vi "CreateOrOpenProject.vi"(8 "error in (no error)":errorcluster, 11 "ProjectPath":path) -> (0 "error out":errorcluster)   [LabVIEW 2013, in "ProjectHandler.lvlib"]
uses:
  ProjectHandler.lvlib
  RefNums.vi
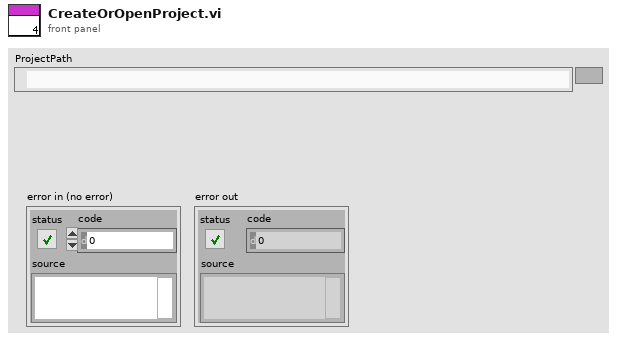
[diagram p1: front panel]
types:
  T1 = cluster{"App":refnum<vi>, "Project":refnum<vi>, "My Computer":refnum<vi>}
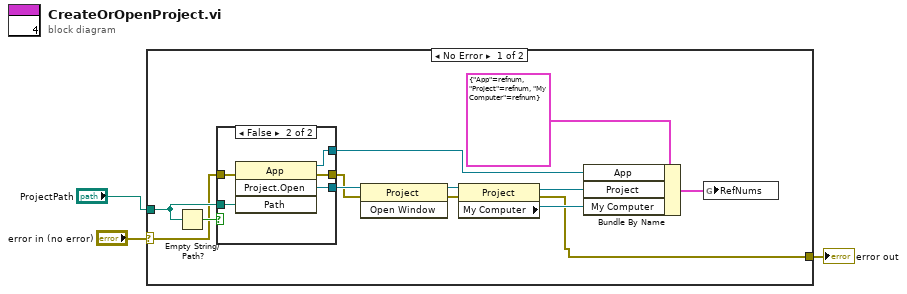
[diagram p0: block diagram]
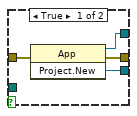
[diagram p2: hidden frame]
diagram:
  n1 = case shown="No Error" "error in (no error)" {
    selector: "error in (no error)" -> [w10 w26]
    tunnel: "ProjectPath" -> [w11 _]
    tunnel: [w4 w26] -> w1
    frame No Error {
      n2 = Empty String/Path?(string/path=w11) -> (empty?=w16:bool)
      n3 = case shown="False" w16 {
        tunnel: w10 -> [w20 w21]
        tunnel: [w19 w24] -> w14
        tunnel: [w18 w23] -> w13
        tunnel: w11 -> [_ w25]
        tunnel: [w17 w22] -> w8
        frame True {
          n4 = invoke class="App" method="Project.New"(error in=w20) -> (reference out=w17:refnum<vi>, error out=w18:errorcluster, "Project:New"=w19:refnum<vi>)  [unwired: 2 in]
        }
        frame False {
          n5 = invoke class="App" method="Project.Open"(error in=w21, "Path"=w25) -> (reference out=w22:refnum<vi>, error out=w23:errorcluster, "Project:Open"=w24:refnum<vi>)  [unwired: 2 in, 1 out]
        }
      }
      n6 = invoke class="Project" method="Open Window"(reference=w14, error in=w13) -> (reference out=w12:refnum<vi>, error out=w15:errorcluster)  [unwired: 1 in, 1 out]
      n7 = property class="Project"(reference=w12, error in=w15) -> (reference out=w7:refnum<vi>, error out=w4:errorcluster, "My Computer"=w6:refnum<vi>)
      n8 = Bundle By Name(cluster=T1 {"App"=refnum, "Project"=refnum, "My Computer"=refnum} ("RefNums"), "App"=w8, "Project"=w7, "My Computer"=w6) -> (w5:T1)
      n9 = global write "RefNums.vi" "RefNums"(w5) -> ()
    }
    frame Error {
    }
  }
  "error out" <- w1
